vi "Read_CoreCluster.vi"(8 "Error In":errorcluster, 11 "EVE in":refnum<class "EVE.lvclass">) -> (0 "Error out":errorcluster, 2 "Core":T1, 3 "EVE out":refnum<class "EVE.lvclass">)   [LabVIEW 2013, in "EVE.lvclass"]
uses:
  EVE.lvclass
  CoreCluster.ctl
  030 - EVENTS/01 - ToHmiScheduler/ToHmiScheduler.ctl
  030 - EVENTS/01 - ToHmiScheduler/ToHmiSchedulerCommand.ctl
  030 - EVENTS/03 - ToMessageHandlerProcess/ToMessageHandlerEvent.ctl
  030 - EVENTS/03 - ToMessageHandlerProcess/enumMessageCriticity.ctl
  030 - EVENTS/02 - ToScreens/ToScreen.ctl
  030 - EVENTS/02 - ToScreens/ToScreensCommand.ctl
  030 - EVENTS/04 - ToAllProcesses/ToAllProcessesEvent.ctl
  030 - EVENTS/04 - ToAllProcesses/EnumToAllProcessesCommand.ctl
  030 - EVENTS/06 - ToProcess/ToProcess.ctl
  030 - EVENTS/06 - ToProcess/ToProcess_EnumCommand.ctl
  030 - EVENTS/00 - ToSplashScreen/ToSplashScreen.ctl
  030 - EVENTS/05 - FromProcesses/FromProcessEvent.ctl
  030 - EVENTS/05 - FromProcesses/FromProcessesEventType.ctl
  Messages/Messages.lvclass
  Core_Processes-Cluster.ctl
  100_PROCESS/Class/Process/Process.lvclass
  EVE.lvclass/EVE.ctl
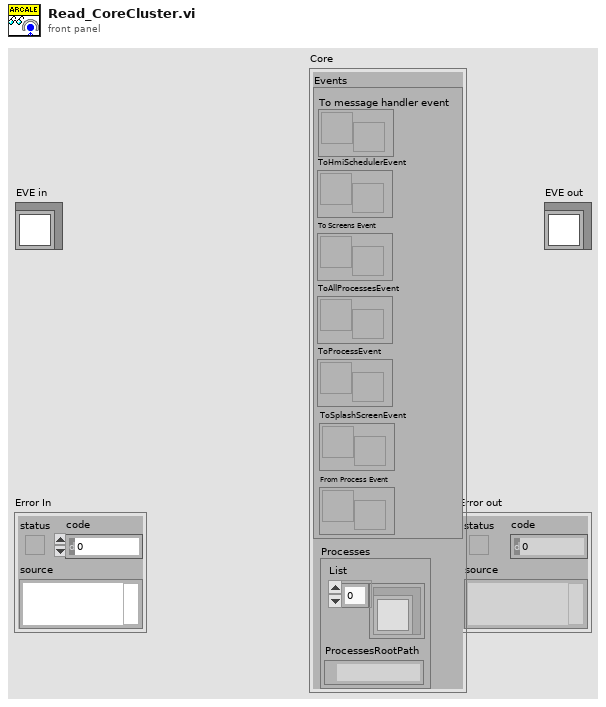
[diagram p1: front panel]
types:
  T1 = typedef "EVE.lvclass/CoreCluster.ctl" = cluster{"Events":cluster{"ToHmiSchedulerEvent":refnum<user-event>, "To Screens Event":refnum<user-event>, "ToAllProcessesEvent":refnum<user-event>, "ToProcessEvent":refnum<user-event>, "ToSplashScreenEvent":refnum<user-event>, "From Process Event":refnum<user-event>, "To message handler event":refnum<user-event>}, "Processes":T2}
  T2 = typedef "EVE.lvclass/Core_Processes-Cluster.ctl" = cluster{"List":refnum<class "Process.lvclass">[], "ProcessesRootPath":path}
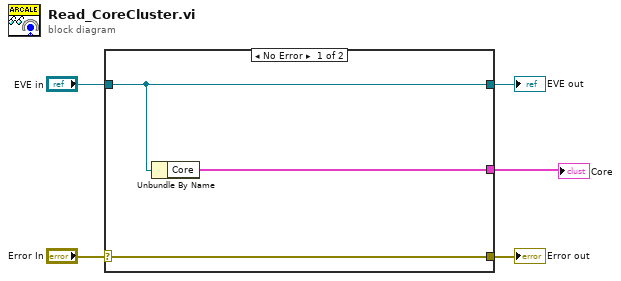
[diagram p0: block diagram]
diagram:
  n1 = case shown="No Error" "Error In" {
    selector: "Error In" -> [w8 w9]
    tunnel: [w8 w9] -> w4
    tunnel: [w7 w10] -> w2
    tunnel: "EVE in" -> [w7 w10]
    tunnel: [w6 _] -> w1
    frame No Error {
      n2 = Unbundle By Name(w7) -> ("Core"=w6:T1)
    }
    frame Error {
    }
  }
  "Error out" <- w4
  "EVE out" <- w2
  "Core" <- w1
